vi "Do.vi"(8 "error in":errorcluster, 11 "CAN Task in":refnum<class "CANopen Task Actor.lvclass">) -> (0 "error out":errorcluster, 3 "CAN Task out":refnum<class "CANopen Task Actor.lvclass">)   [LabVIEW 2024, in "CANopen Task Actor.lvlib" / "CANopen Task Actor.lvclass"]
uses:
  CANopen Task Actor.lvclass
  CANopen Task Actor.lvclass/CANopen Task Actor.ctl
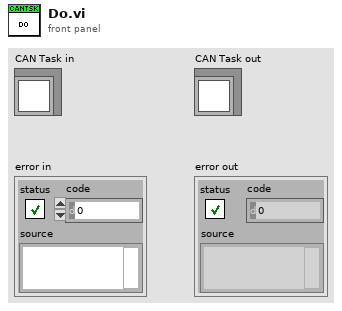
[diagram p1: front panel]
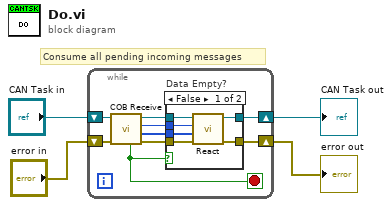
[diagram p0: block diagram]
diagram:
  # "Consume all pending incoming messages"
  n1 = while {
    shift-right: [w7] -> w2
    shift-left: "error in" -> [w13]
    shift-right: [w6] -> w1
    shift-left: "CAN Task in" -> [w12]
    stop <- w5 stop-if-true
    n2 = call "COB Receive.vi"("error in"=w13, "CAN Task in"=w12) -> ("error out"=w8:errorcluster, "Data"=w9:u8[], "COB ID"=w10:u32, "CAN Task out"=w11:refnum<class "CANopen Task Actor.lvclass">, "No Data?"=w5:bool)  [unwired: 5 in]
    n3 = case "Data Empty?" shown="False" w5 {
      tunnel: w11 -> [w19 w20]
      tunnel: w10 -> [w18 _]
      tunnel: w9 -> [w17 _]
      tunnel: w8 -> [w16 w21]
      tunnel: [w15 w21] -> w7
      tunnel: [w14 w20] -> w6
      frame False {
        n4 = call "React.vi"("error in"=w16, "Data"=w17, "COB ID"=w18, "CAN Task in"=w19) -> ("error out"=w15:errorcluster, "CAN Task out"=w14:refnum<class "CANopen Task Actor.lvclass">)  [unwired: 6 in]
      }
      frame True {
      }
    }
  }
  "error out" <- w2
  "CAN Task out" <- w1
